vi "Initialize1.vi"(8 "error in (no error)":errorcluster, 9 "Reset (True)":bool=TRUE, 10 "ID Query (True)":bool=TRUE, 11 "VISA resource name":refnum<visa-resource-name>) -> (0 "error out":errorcluster, 2 "read buffer":string, 3 "VISA resource name out":refnum<visa-resource-name>)   [LabVIEW 2015, in "Agilent 3446X Series1.lvlib"]
doc: "Establishes communication with the instrument and optionally performs an instrument identification query and/or an instrument reset. It also places the instrument in a default state needed for other instrument driver operations. Therefore, call this VI before calling other instrument driver VIs for this instrument. Generally, you need to call the Initialize VI only once at the beginning of an application."
uses:
  Agilent 3446X Series1.lvlib
panel:
  # "(c) 2013 National Instruments.  ALL RIGHTS RESERVED."
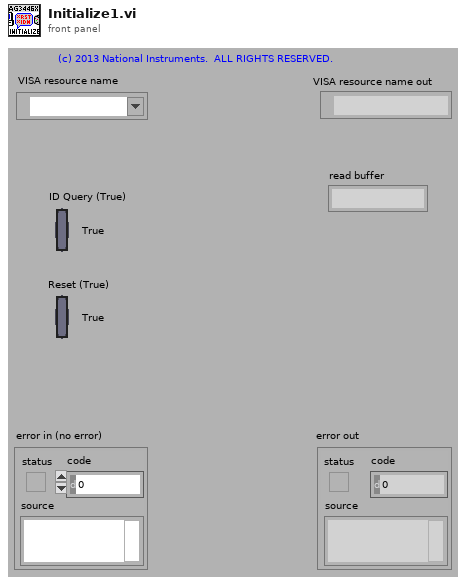
[diagram p1: front panel]
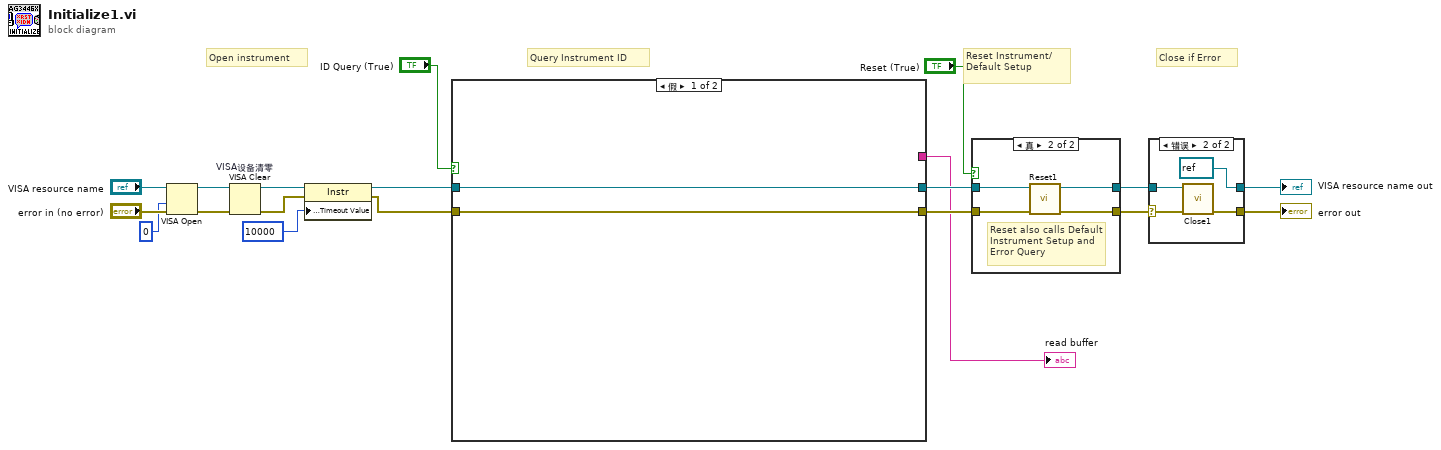
[diagram p0: block diagram]
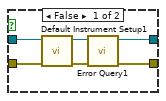
[diagram p3: hidden frame]
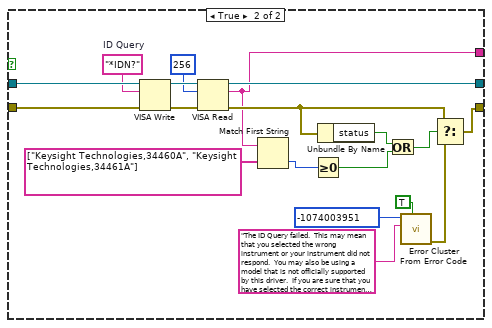
[diagram p4: hidden frame]
diagram:
  # "Close if Error"
  # "Query Instrument ID"
  # "Reset Instrument/\nDefault Setup"
  # "Open instrument"
  n1 = VISA Open(access mode=u32 0, error in (no error)="error in (no error)", VISA resource name="VISA resource name") -> (VISA resource name=w11:refnum<visa-resource-name>, error out=w10:errorcluster)  [unwired: 2 out]
  n2 = VISA Clear "VISA设备清零"(VISA resource name=w11, error in (no error)=w10) -> (VISA resource name out=w9:refnum<visa-resource-name>, error out=w8:errorcluster)
  n3 = property class="Instr"(reference=w9, error in=w8, "General Settings:Timeout Value"=u32 10000) -> (reference out=w3:refnum<visa-resource-name>, error out=w2:errorcluster)
  n4 = case shown="假" "ID Query (True)" {
    tunnel: [w20 w40] -> w18
    tunnel: [w21 w37] -> w19
    tunnel: w3 -> [w21 w38]
    tunnel: w2 -> [w20 w39]
    tunnel: [_ w22] -> w1
    frame False {
    }
    frame True {
      w33 = "*IDN?"  # ID Query
      n5 = VISA Write(VISA resource name=w38, write buffer=w33, error in (no error)=w39) -> (VISA resource name out=w36:refnum<visa-resource-name>, error out=w35:errorcluster)  [unwired: 1 out]
      n6 = VISA Read(VISA resource name=w36, byte count=u32 256, error in (no error)=w35) -> (VISA resource name out=w37:refnum<visa-resource-name>, read buffer=w22:string, error out=w28:errorcluster)  [unwired: 1 out]
      n7 = Match First String(2:string[] ["Keysight Technologies,34460A", "Keysight Technologies,34461A"] ("string array"), 3:w22) -> (0:w23:i32)  [unwired: 1 out]
      n8 = Greater Or Equal To 0?(x=w23) -> (x >= 0?=w26:bool)
      n9 = Unbundle By Name(w28) -> ("status"=w27:bool)
      n10 = Or(x=w27, y=w26) -> (x .or. y?=w25:bool)
      n11 = call <vilib>:"Error Cluster From Error Code.vi"("show call chain? (False)"=TRUE, "error message (\"\")"="The ID Query failed.  This may mean that you selected the wrong instrument or your instrument did not respond.  You may also be using a model that is not officially supported by this driver.  If you are sure that you have selected the correct instrument and it is responding, try disabling the ID Query." ("Source (VI Name)"), "error code (0)"=-1074003951 ("Code")) -> ("error out"=w32:errorcluster)  [unwired: 1 in, 5 out]
      n12 = Select(t=w28, s=w25, f=w32) -> (s? t:f=w40:errorcluster)
    }
  }
  "read buffer" <- w1
  n13 = case shown="真" "Reset (True)" {
    tunnel: w18 -> [w45 w47]
    tunnel: [w42 w50] -> w4
    tunnel: w19 -> [w46 w48]
    tunnel: [w43 w49] -> w5
    frame False {
      n14 = call "Default Instrument Setup1.vi"("error in (no error)"=w45, "VISA resource name"=w46) -> ("error out"=w41:errorcluster, "VISA resource name out"=w44:refnum<visa-resource-name>)  [unwired: 8 out]
      n15 = call "Error Query1.vi"("error in (no error)"=w41, "VISA resource name"=w44) -> ("error out"=w42:errorcluster, "VISA resource name out"=w43:refnum<visa-resource-name>)  [unwired: 8 out]
    }
    frame True {
      # "Reset also calls Default Instrument Setup and Error Query"
      n16 = call "Reset1.vi"("error in (no error)"=w47, "VISA resource name"=w48) -> ("error out"=w50:errorcluster, "VISA resource name out"=w49:refnum<visa-resource-name>)  [unwired: 8 out]
    }
  }
  n17 = case shown="错误" w4 {
    selector: w4 -> [w51 w54]
    tunnel: w5 -> [w52 w55]
    tunnel: [w52 refnum<visa-resource-name> refnum ("VISA resource name out")] -> w7
    tunnel: [w51 w56] -> w6
    frame No Error {
    }
    frame Error {
      n18 = call "Close1.vi"("error in (no error)"=w54, "VISA resource name"=w55) -> ("error out"=w56:errorcluster)  [unwired: 9 out]
    }
  }
  "VISA resource name out" <- w7
  "error out" <- w6
